vi "Parse YAML.vi"(8 "error in (no error)":errorcluster, 10 "YAML String":string, 11 "YAML Parser in":refnum<class "YAML Parser.lvclass">) -> (0 "error out":errorcluster, 3 "YAML Parser out":refnum<class "YAML Parser.lvclass">)   [LabVIEW 2015, in "YAML Parser.lvclass"]
uses:
  YAML Parser.lvclass
  YAML Parser.lvclass/YAML Parser.ctl
  YAML Parser.lvlib
panel:
  out "Remaining String":string
  out "Data out":variant
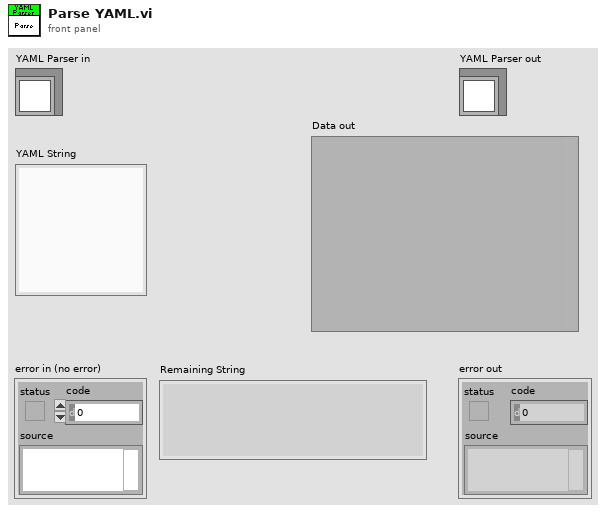
[diagram p1: front panel]
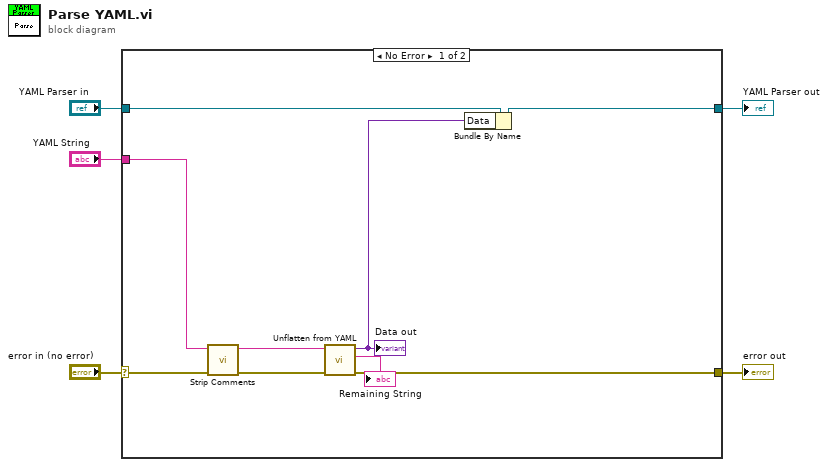
[diagram p0: block diagram]
diagram:
  n1 = case shown="No Error" "error in (no error)" {
    selector: "error in (no error)" -> [w13 w16]
    tunnel: [w8 w16] -> w4
    tunnel: [w11 w15] -> w2
    tunnel: "YAML Parser in" -> [w14 w15]
    tunnel: "YAML String" -> [w12 _]
    frame No Error {
      n2 = call "Strip Comments.vi"("error in (no error)"=w13, "String"=w12) -> ("error out"=w10:errorcluster, "String out"=w9:string)  [unwired: 7 in, 1 out]
      n3 = call "Unflatten from YAML.vi"("error in (no error)"=w10, "YAML String"=w9) -> ("error out"=w8:errorcluster, "Remaining String"=→"Remaining String":string, "Anything"=w7:variant)  [unwired: 7 in]
      "Data out" <- w7
      n4 = Bundle By Name(cluster=w14, "Data"=w7) -> (w11:refnum<class "YAML Parser.lvclass">)
    }
    frame Error {
    }
  }
  "error out" <- w4
  "YAML Parser out" <- w2
